vi "Read NET_MultipartContent.vi"(8 "error in (no error)":errorcluster, 11 "HttpContent_Multipart in":refnum<class "HttpContent_Multipart.lvclass">) -> (0 "error out":errorcluster, 2 "NET_MultipartContent":refnum<k24>, 3 "HttpContent_Multipart out":refnum<class "HttpContent_Multipart.lvclass">)   [LabVIEW 2018, in "HttpClient_NET.lvlib" / "HttpContent_Multipart.lvclass"]
doc: "<b> </b> <b> </b>\nHttpClient_NET\nJustin Young - Viviota\nCopyright (c) 2021\nLicense: BSD"
uses:
  HttpContent_Multipart.lvclass
  C:/Viviota/Projects/R&D/__OpenSource/VIV_HTTP_REST_NET/HttpContent/HttpContent.lvclass
  System.Net.Http
  HttpContent/HttpContent.lvclass/HttpContent.ctl
  HttpContent/HttpContent.lvclass
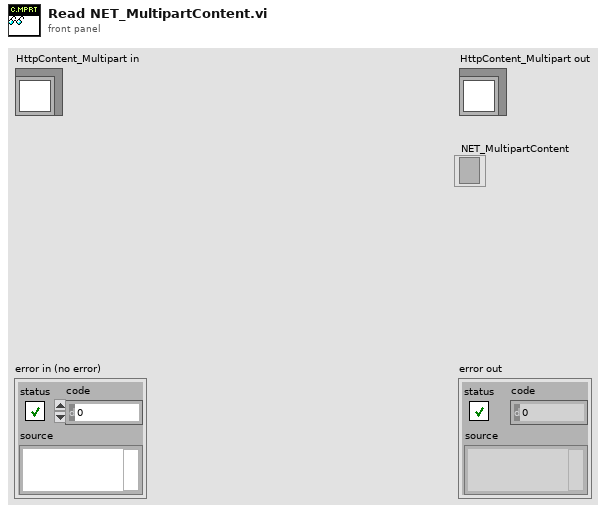
[diagram p1: front panel]
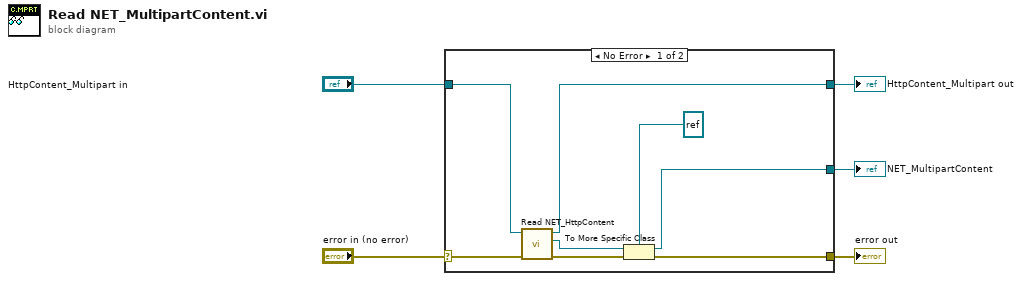
[diagram p0: block diagram]
diagram:
  n1 = case shown="No Error" "error in (no error)" {
    selector: "error in (no error)" -> [w13 w14]
    tunnel: [w12 w14] -> w4
    tunnel: [w7 w15] -> w2
    tunnel: "HttpContent_Multipart in" -> [w8 w15]
    tunnel: [w11 _] -> w1
    frame No Error {
      n2 = call "Read NET_HttpContent.vi"("error in (no error)"=w13, "HttpContent in"=w8) -> ("error out"=w9:errorcluster, "NET_HttpContent"=w6:refnum<k24>, "HttpContent out"=w7:refnum<class "HttpContent_Multipart.lvclass">)  [unwired: 7 in]
      n3 = To More Specific Class(target class=refnum<k24> refnum ("NET_MultipartContent"), reference=w6, error in=w9) -> (specific class reference=w11:refnum<k24>, error out=w12:errorcluster)
    }
    frame Error {
    }
  }
  "error out" <- w4
  "HttpContent_Multipart out" <- w2
  "NET_MultipartContent" <- w1
